vi "zadanie_4.vi"() -> ()   [LabVIEW 2020]
panel:
  out "Waveform Graph":i32[](graph)
  in  "stop":bool
  out "F(n)":u32
  in  "n":dbl
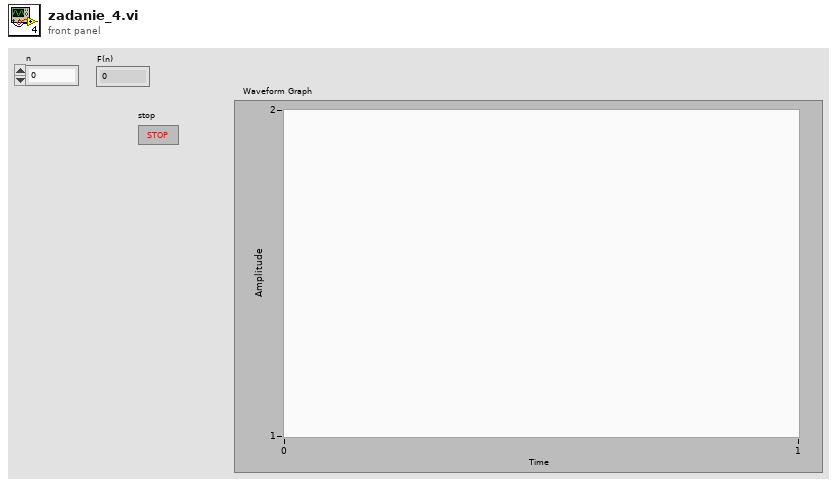
[diagram p1: front panel]
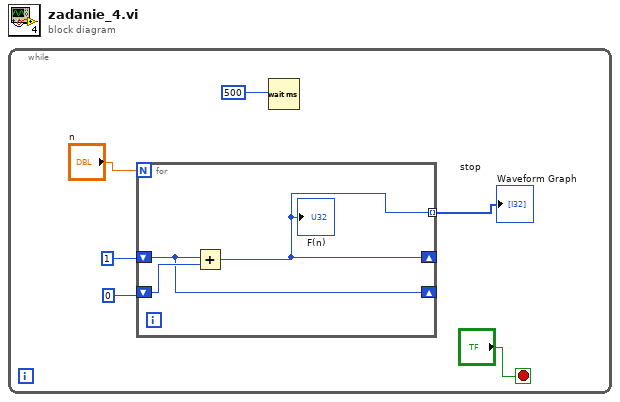
[diagram p0: block diagram]
diagram:
  n1 = while {
    stop <- "stop" stop-if-true
    n2 = for {
      N: "n" -> [_]
      shift-right: [w7] -> _
      shift-left: 1 -> [w8]
      shift-right: [w8] -> _
      shift-left: 0 -> [w9]
      tunnel: [w7] -> w1 mode=indexing
      n3 = Add(x=w8, y=w9) -> (x+y=w7:i32)
      "F(n)" <- w7
    }
    "Waveform Graph" <- w1
    n4 = Wait (ms)(milliseconds to wait=500) -> ()  [unwired: 1 out]
  }
